vi "MoveAI.vi"(7 "ReturnHome(F)":bool, 8 "error in (no error)":errorcluster, 10 "Ball":refnum<class "PongBall.lvclass">, 11 "PongPanel in":refnum<class "PongPanel.lvclass">) -> (0 "error out":errorcluster, 3 "PongPanel out":refnum<class "PongPanel.lvclass">)   [LabVIEW 2019, in "RT_Game.lvlib" / "PongPanel.lvclass"]
uses:
  PongPanel.lvclass
  C:/Users/FreshBob/Dropbox/VIs/myRIO_GameConsole/RT/RT_Game/GameObject/GameObject.lvclass
  PongBall/PongBall.lvclass
  GameObject/GameObject.lvclass/GameObject.ctl
  PongPanel.lvclass/PongPanel.ctl
  GameObject/Read Velocity.vi
  GameObject/GameObject.lvclass
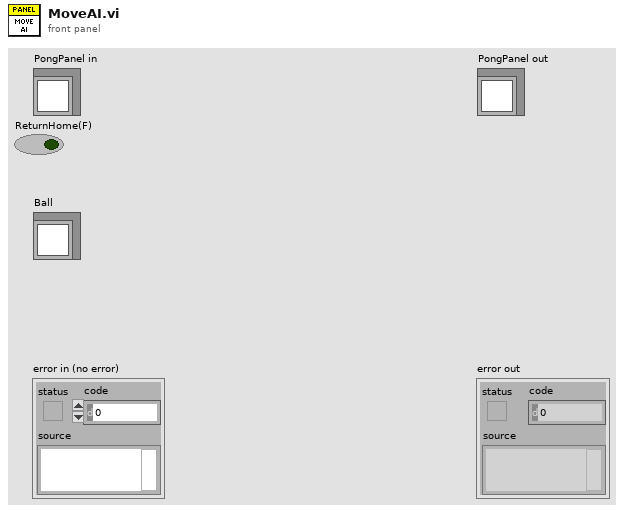
[diagram p1: front panel]
types:
  T1 = typedef "Velocity.ctl" = cluster{"x":dbl, "y":dbl}
  T2 = typedef "RT_Game.lvlib/Game.lvclass/Coordinate.ctl" = cluster{"x":dbl, "y":dbl}
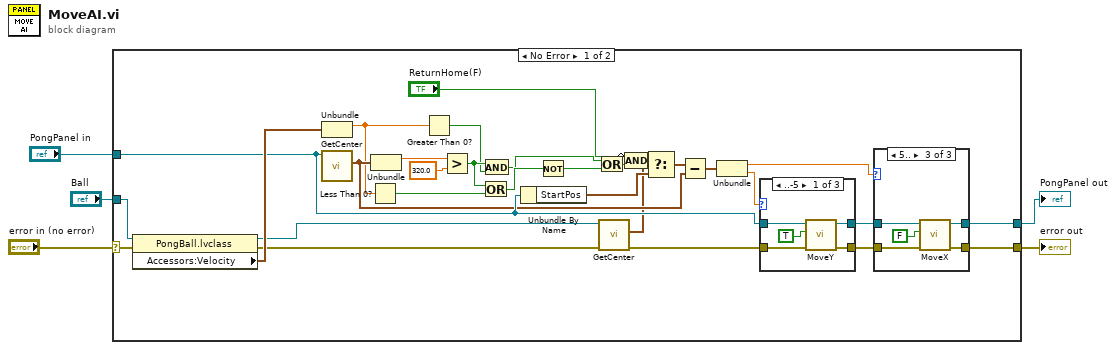
[diagram p0: block diagram]
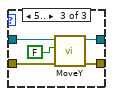
[diagram p3: hidden frame]
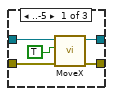
[diagram p4: hidden frame]
diagram:
  n1 = case shown="No Error" "error in (no error)" {
    selector: "error in (no error)" -> [w35 w61]
    tunnel: [w34 w61] -> w4
    tunnel: [w33 w60] -> w2
    tunnel: "PongPanel in" -> [w30 w60]
    tunnel: "Ball" -> [w32 _]
    frame No Error {
      n2 = property class="PongBall.lvclass"(reference=w32, error in=w35) -> (reference out=w28:refnum<class "PongBall.lvclass">, error out=w29:errorcluster, "Accessors:Velocity"=w31:T1)
      n3 = Unbundle(w31) -> ("x"=w9:dbl)  [unwired: 1 out]
      n4 = call "GetCenter.vi"("GameObject in"=w30) -> ("center_pos"=w12:T2)  [unwired: 8 in, 2 out]
      n5 = Less Than 0?(x=w9) -> (x < 0?=w8:bool)
      n6 = Unbundle(w12) -> ("x"=w27:dbl)  [unwired: 1 out]
      n7 = Greater Than 0?(x=w9) -> (x > 0?=w24:bool)
      n8 = Greater?(x=w27, y=320.0) -> (0:w25:bool)
      n9 = Or(x=w25, y=w8) -> (x .or. y?=w23:bool)
      n10 = And(x=w25, y=w24) -> (x .and. y?=w21:bool)
      n11 = Unbundle By Name(w30) -> ("StartPos"=w13:T2)
      n12 = Not(x=w23) -> (.not. x?=w22:bool)
      n13 = Or(x=w21, y=w22) -> (x .or. y?=w14:bool)
      n14 = call "GetCenter.vi"("error in (no error)"=w29, "GameObject in"=w28) -> ("error out"=w11:errorcluster, "center_pos"=w10:T2)  [unwired: 7 in, 1 out]
      n15 = Compound Arithmetic op=AND(invert "ReturnHome(F)", w14) -> (w7:bool)
      n16 = Select(t=w10, s=w7, f=w13) -> (s? t:f=w15:T2)
      n17 = Subtract(x=w15, y=w12) -> (x-y=w18:T2)
      n18 = Unbundle(w18) -> ("x"=w16:dbl, "y"=w17:dbl)
      n19 = case shown="..-5" w17 {
        tunnel: [w39 w41 w47] -> w20
        tunnel: [w37 w42 w46] -> w19
        tunnel: w11 -> [w40 w41 w45]
        tunnel: w30 -> [w38 w42 w44]
        frame ..-5 {
          n20 = call "MoveY.vi"("error in (no error)"=w40, "Up?"=TRUE, "PongPanel in"=w38) -> ("error out"=w39:errorcluster, "PongPanel out"=w37:refnum<class "PongPanel.lvclass">)  [unwired: 7 in]
        }
        frame 0, Default {
        }
        frame 5.. {
          n21 = call "MoveY.vi"("error in (no error)"=w45, "Up?"=FALSE, "PongPanel in"=w44) -> ("error out"=w47:errorcluster, "PongPanel out"=w46:refnum<class "PongPanel.lvclass">)  [unwired: 7 in]
        }
      }
      n22 = case shown="5.." w16 {
        tunnel: w20 -> [w52 w53 w59]
        tunnel: [w51 w53 w58] -> w34
        tunnel: w19 -> [w50 w54 w57]
        tunnel: [w49 w54 w56] -> w33
        frame ..-5 {
          n23 = call "MoveX.vi"("error in (no error)"=w52, "Left?"=TRUE, "PongPanel in"=w50) -> ("error out"=w51:errorcluster, "PongPanel out"=w49:refnum<class "PongPanel.lvclass">)  [unwired: 7 in]
        }
        frame 0, Default {
        }
        frame 5.. {
          n24 = call "MoveX.vi"("error in (no error)"=w59, "Left?"=FALSE ("Up?"), "PongPanel in"=w57) -> ("error out"=w58:errorcluster, "PongPanel out"=w56:refnum<class "PongPanel.lvclass">)  [unwired: 7 in]
        }
      }
    }
    frame Error {
    }
  }
  "error out" <- w4
  "PongPanel out" <- w2
